vi "Compare Modules.vi"(8 "error in (no error)":errorcluster, 10 "All Mods":refnum<k21>[](array[refnum]), 11 "RSI Modules in":T1[](array[typedef]) {"Module Config Data"."Config Block Data Refs"."Data Reference" format="%.0x"; "Output Data"."Output Block Data Refs"."Data Reference" format="%.0x"; "Input Data"."Input Block Data Refs"."Data Reference" format="%.0x"; "VS ref" format="%.0x"}) -> (0 "error out":errorcluster, 3 "RSI Modules out":T1[](array[typedef]) {"Module Config Data"."Config Block Data Refs"."Data Reference" format="%.0x"; "Output Data"."Output Block Data Refs"."Data Reference" format="%.0x"; "Input Data"."Input Block Data Refs"."Data Reference" format="%.0x"; "VS ref" format="%.0x"})   [LabVIEW 2011, in "Scan Engine Custom Device.lvlib"]
uses:
  Scan Engine Custom Device.lvlib
  Type Defs/RSI Module Data.ctl
  <vilib>/NI Veristand/Custom Device API/Custom Device Item Ref.ctl
  Modules.lvlibp/RSI Module/RSI Module.lvclass
  Modules.lvlibp/RSI Module/Module Models.ctl
  Modules.lvlibp/RSI Module/Channel Type.ctl
  Type Defs/Input Data.ctl
  <vilib>/NI Veristand/Custom Device API/Block Data Reference.ctl
  <vilib>/NI Veristand/Custom Device API/Data Reference.ctl
  Type Defs/Output Data.ctl
  Type Defs/Module Config Data.ctl
  Type Defs/Mixed IO.ctl
  Globals/Error Strings.vi
  Program Files (x86)/National Instruments/LabVIEW 2011/resource/objmgr/cRIO.rc
  <vilib>/NI Veristand/Custom Device API/Custom Device API.lvlib
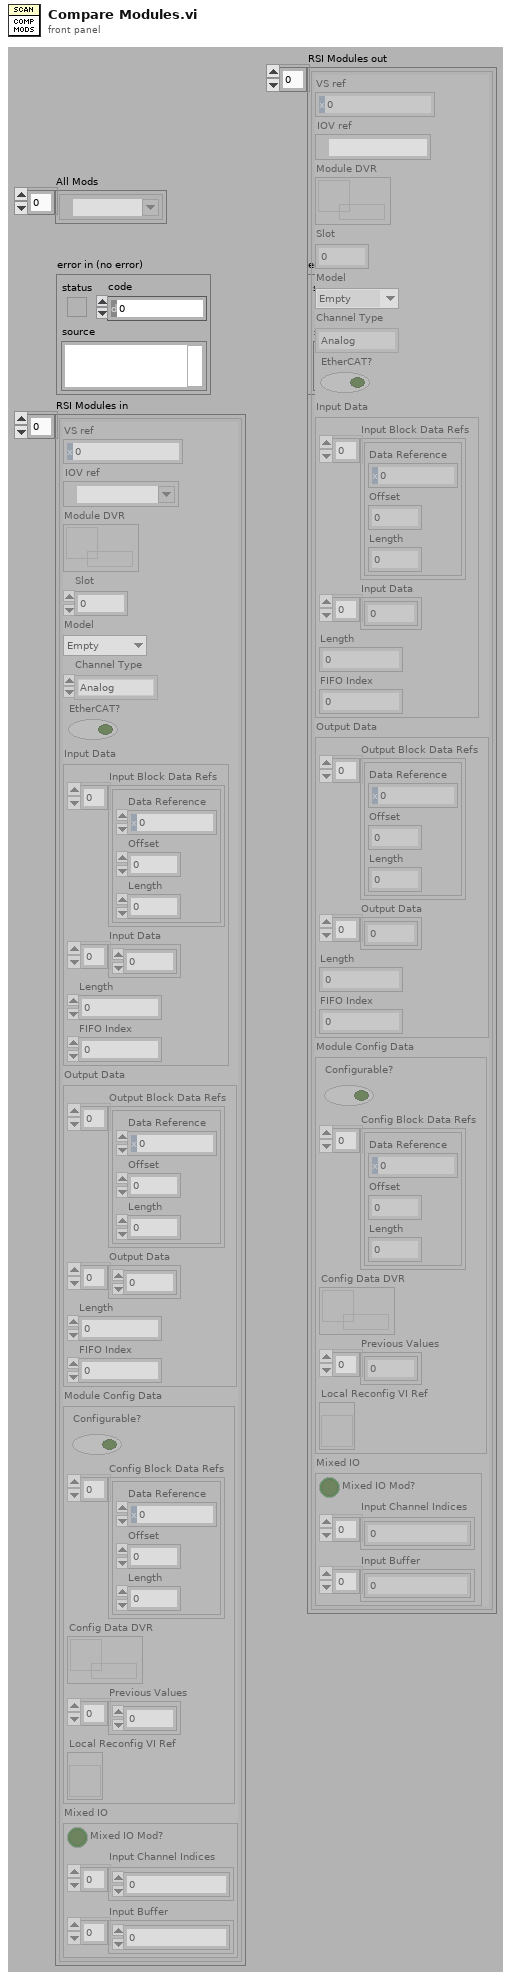
[diagram p1: front panel]
types:
  T1 = typedef "Scan Engine Custom Device.lvlib/RSI Module Data.ctl" = cluster{"VS ref":T2, "IOV ref":refnum<k21>, "Module DVR":refnum<data-value>, "Slot":u32, "Model":T3, "Channel Type":T4, "EtherCAT?":bool, "Input Data":T5, "Output Data":T8, "Module Config Data":T9, "Mixed IO":T10}
  T2 = typedef "Custom Device API.lvlib/Custom Device Item Ref.ctl" = u64
  T3 = typedef "Modules.lvlibp/RSI Module.lvclass/Module Models.ctl" = enum16{"Empty", "NI 9201", "NI 9203", "NI 9205", "NI 9206", "NI 9207", "NI 9208", "NI 9211", "NI 9213", "NI 9214", "NI 9215", "NI 9217", "NI 9219", "NI 9221", "NI 9225", "NI 9227", "NI 9229", "NI 9233", "NI 9234", "NI 9235", "NI 9236", "NI 9237", "NI 9239", "NI 9263", "NI 9264", "NI 9265", "NI 9269", "NI 9375", "NI 9401", "NI 9402", "NI 9403", "NI 9411", "NI 9421", "NI 9422", "NI 9423", "NI 9425", "NI 9426", "NI 9435", "NI 9472", "NI 9474", "NI 9475", "NI 9476", "NI 9477", "NI 9478", "NI 9481", "NI 9482", "NI 9485"}
  T4 = typedef "Modules.lvlibp/RSI Module.lvclass/Channel Type.ctl" = enum16{"Analog", "Digital"}
  T5 = typedef "Scan Engine Custom Device.lvlib/Input Data.ctl" = cluster{"Input Block Data Refs":T6[], "Input Data":dbl[], "Length":i32, "FIFO Index":i32}
  T6 = typedef "Custom Device API.lvlib/Block Data Reference.ctl" = cluster{"Data Reference":T7, "Offset":i32, "Length":i32}
  T7 = typedef "Custom Device API.lvlib/Data Reference.ctl" = i32
  T8 = typedef "Scan Engine Custom Device.lvlib/Output Data.ctl" = cluster{"Output Block Data Refs":T6[], "Output Data":dbl[], "Length":i32, "FIFO Index":i32}
  T9 = typedef "Scan Engine Custom Device.lvlib/Module Config Data.ctl" = cluster{"Configurable?":bool, "Config Block Data Refs":T6[], "Config Data DVR":refnum<data-value>, "Previous Values":dbl[], "Local Reconfig VI Ref":refnum<vi>}
  T10 = typedef "Scan Engine Custom Device.lvlib/Mixed IO.ctl" = cluster{"Mixed IO Mod?":bool, "Input Channel Indices":i32[], "Input Buffer":dbl[]}
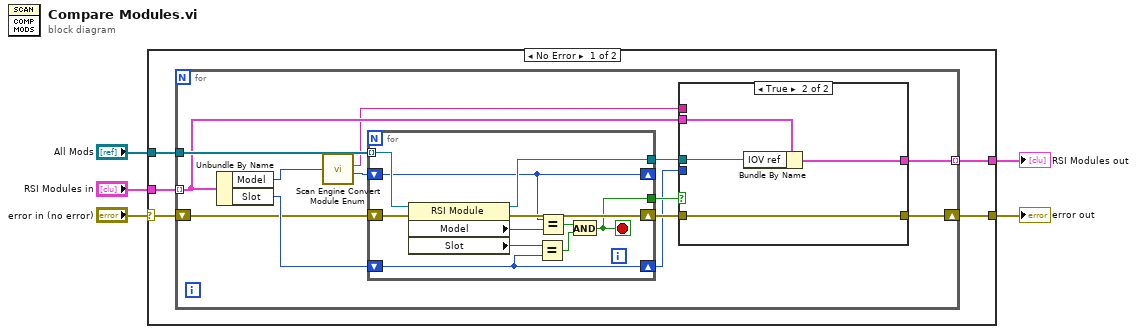
[diagram p0: block diagram]
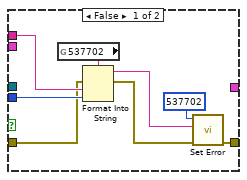
[diagram p2: hidden frame]
diagram:
  n1 = case shown="No Error" "error in (no error)" {
    selector: "error in (no error)" -> [w10 w47]
    tunnel: [w9 w47] -> w4
    tunnel: "RSI Modules in" -> [w7 _]
    tunnel: "All Mods" -> [w8 _]
    tunnel: [w6 _] -> w1
    frame No Error {
      n2 = for {
        tunnel: w8 -> [w23]
        shift-right: [w20] -> w9
        shift-left: w10 -> [w13]
        tunnel: w7 -> [w17] mode=indexing
        tunnel: [w16] -> w6 mode=indexing
        n3 = Unbundle By Name(w17) -> ("Model"=w15:T3, "Slot"=w14:u32)
        n4 = call "Scan Engine Convert Module Enum.vi"("Module"=w15) -> ("Model Number"=w18:u32, "Module Name"=w12:string)  [unwired: 2 in]
        n5 = for {
          tunnel: w23 -> [w46] mode=indexing
          shift-right: [w44] -> w21
          shift-left: w13 -> [w45]
          tunnel: [w39] -> w22
          tunnel: [w43] -> w19
          shift-right: [w42] -> _
          shift-left: w18 -> [w42]
          shift-right: [w36] -> w11
          shift-left: w14 -> [w36]
          stop <- w39 stop-if-true
          n6 = property class="RSI Module"(reference=w46, error in=w45) -> (reference out=w43:refnum<k21>, error out=w44:errorcluster, "Model"=w37:u32, "Slot"=w38:u32)
          n7 = Equal?(x=w38, y=w36) -> (x = y?=w41:bool)
          n8 = Equal?(x=w42, y=w37) -> (x = y?=w40:bool)
          n9 = And(x=w40, y=w41) -> (x .and. y?=w39:bool)
        }
        n10 = case shown="True" w22 {
          tunnel: [w30 w33] -> w20
          tunnel: w21 -> [w25 w33]
          tunnel: w19 -> [_ w34]
          tunnel: [_ w35] -> w16
          tunnel: w17 -> [_ w32]
          tunnel: w12 -> [w28 _]
          tunnel: w11 -> [w27 _]
          frame False {
            n11 = global read "Error Strings.vi" "537702"() -> (w29:string)
            n12 = Format Into String(format string=w29, error in=w25, w28, w27) -> (resulting string=w26:string, error out=w24:errorcluster)  [unwired: 1 in]
            n13 = call "Set Error.vi"("error in (no error)"=w24, "Message"=w26, "Code"=537702) -> ("error out"=w30:errorcluster)  [unwired: 8 in]
          }
          frame True {
            n14 = Bundle By Name(cluster=w32, "IOV ref"=w34) -> (w35:T1)
          }
        }
      }
    }
    frame Error {
    }
  }
  "error out" <- w4
  "RSI Modules out" <- w1
